vi "testWDT.vi"() -> ()   [LabVIEW 2010]
panel:
  in  "unit":enum8{"seconds", "minutes"}(ring)
  in  "tick":u8=1 min=1
  out "error_out":errorcluster
  in  "error in (no error)":errorcluster
  out "path out":path
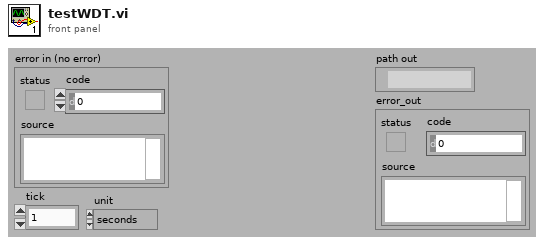
[diagram p1: front panel]
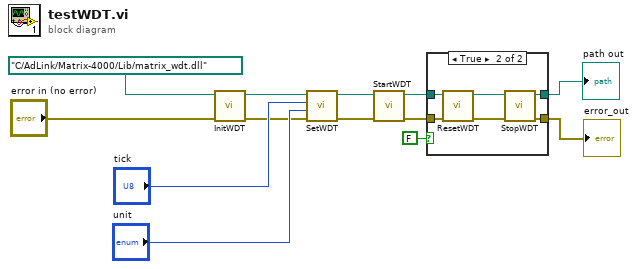
[diagram p0: block diagram]
diagram:
  n1 = call "InitWDT.vi"("error in (no error)"="error in (no error)", "path in"=path "C:/AdLink/Matrix-4000/Lib/matrix_wdt.dll") -> ("error_out"=w9:errorcluster, "path out"=w10:path)  [unwired: 4 in]
  n2 = call "SetWDT.vi"("error in (no error)"=w9, "unit"="unit", "tick"="tick", "path in"=w10) -> ("error out"=w6:errorcluster, "path out"=w7:path)  [unwired: 2 in]
  n3 = call "StartWDT.vi"("error in (no error)"=w6, "path in"=w7) -> ("error out"=w4:errorcluster, "path out"=w5:path)  [unwired: 4 in]
  n4 = case shown="True" FALSE {
    tunnel: w5 -> [w15 w21]
    tunnel: w4 -> [w14 w20]
    tunnel: [w15 w17] -> w3
    tunnel: [w14 w16] -> w2
    frame False {
    }
    frame True {
      n5 = call "ResetWDT.vi"("error in (no error)"=w20, "path in"=w21) -> ("error out"=w18:errorcluster, "path out"=w19:path)  [unwired: 4 in]
      n6 = call "StopWDT.vi"("error in (no error)"=w18, "path in"=w19) -> ("error out"=w16:errorcluster, "path out"=w17:path)  [unwired: 4 in]
    }
  }
  "path out" <- w3
  "error_out" <- w2
